vi "Kinect Acquire.vi"(8 "error in":errorcluster, 11 "Queue in":refnum<queue>) -> (0 "error out":errorcluster, 1 "Timestamp":i32, 2 "Difference\nImage":T1(plugin-control), 3 "Image Out":T1(plugin-control))   [LabVIEW 2011]
uses:
  Kinect Data Cluster.ctl
  <vilib>/vision/NI_Vision_Development_Module.lvlib
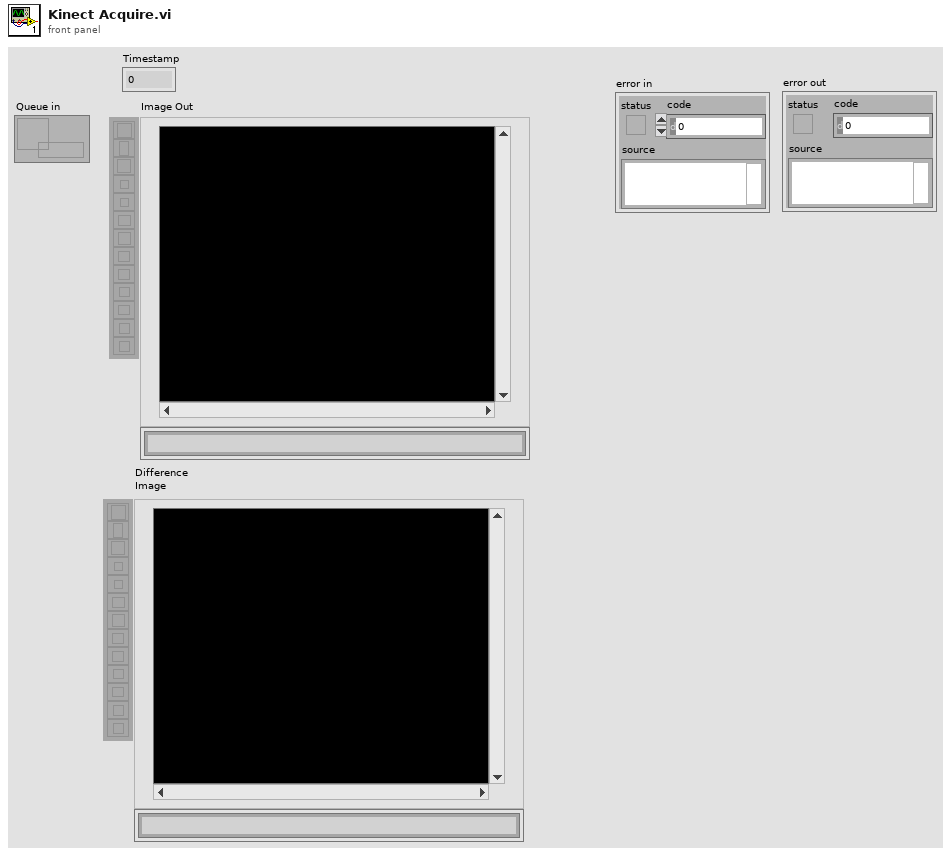
[diagram p1: front panel]
types:
  T1 = typedef "IMAQ Image.ctl" = refnum<image>
  T2 = typedef "Image Type" = u32
  T3 = typedef "Kinect Data Cluster.ctl" = cluster{"1D Depth Data":i16[], "Width":i32, "Height":i32, "Timestamp":i32}
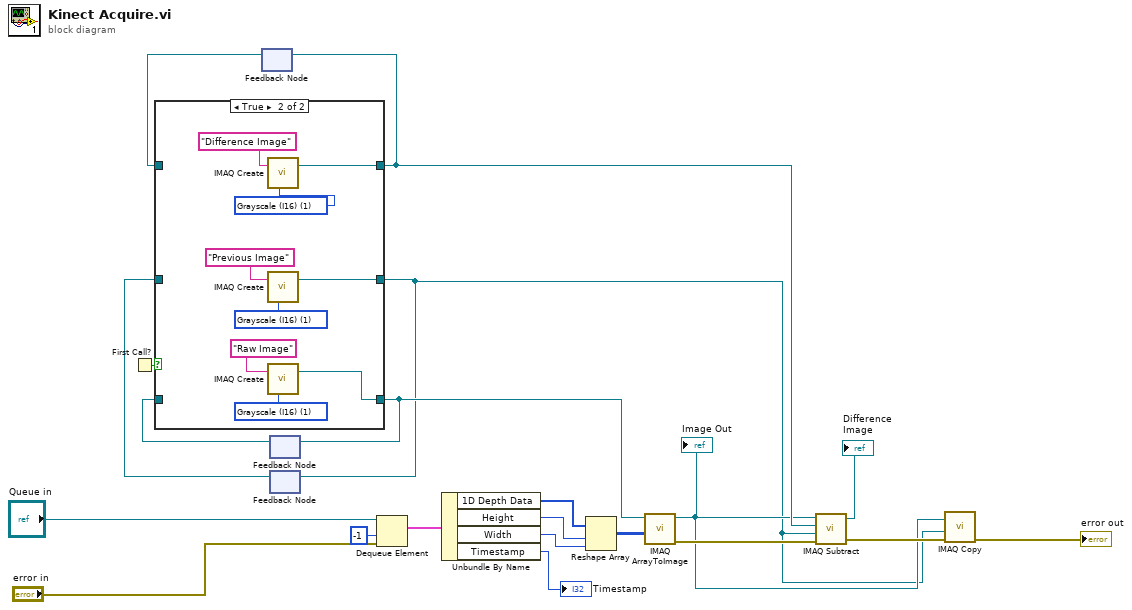
[diagram p0: block diagram]
diagram:
  n1 = First Call?() -> (First Call?: T/F=w8:bool)
  n2 = feedback #1() -> (w16:T1)  [unwired: 1 in]
  n3 = feedback #2() -> (w10:T1)  [unwired: 1 in]
  n4 = feedback #3() -> (w20:T1)  [unwired: 1 in]
  n5 = case shown="True" w8 {
    tunnel: [w24 w31] -> w9
    tunnel: w10 -> [w24 _]
    tunnel: [w23 w29] -> w17
    tunnel: w16 -> [w23 _]
    tunnel: [w22 w25] -> w3
    tunnel: w20 -> [w22 _]
    frame False {
    }
    frame True {
      w27 = T2 1 items=["Grayscale (U8)", "Grayscale (I16)", "Grayscale (SGL)", "Complex (CSG)", "RGB (U32)", "HSL (U32)", "RGB (U64)", "Grayscale (U16)"] ("Image Type")
      w28 = T2 1 items=["Grayscale (U8)", "Grayscale (I16)", "Grayscale (SGL)", "Complex (CSG)", "RGB (U32)", "HSL (U32)", "RGB (U64)", "Grayscale (U16)"] ("Image Type")
      w32 = T2 1 items=["Grayscale (U8)", "Grayscale (I16)", "Grayscale (SGL)", "Complex (CSG)", "RGB (U32)", "HSL (U32)", "RGB (U64)", "Grayscale (U16)"] ("Image Type")
      n6 = call "IMAQ Create"("Image Name"="Difference Image", "Image Type"=w28) -> ("New Image"=w29:T1)  [unwired: 3 in, 1 out]
      n7 = call "IMAQ Create"("Image Name"="Previous Image", "Image Type"=w27) -> ("New Image"=w25:T1)  [unwired: 3 in, 1 out]
      n8 = call "IMAQ Create"("Image Name"="Raw Image", "Image Type"=w32) -> ("New Image"=w31:T1)  [unwired: 3 in, 1 out]
    }
  }
  n9 = feedback-in #1(w17) -> ()
  n10 = feedback-in #2(w9) -> ()
  n11 = feedback-in #3(w3) -> ()
  n12 = Dequeue Element(queue="Queue in", timeout in ms (-1)=-1, error in (no error)="error in") -> (element=w12:T3)  [unwired: 3 out]
  n13 = Unbundle By Name(w12) -> ("1D Depth Data"=w13:i16[], "Height"=w14:i32, "Width"=w15:i32, "Timestamp"=→"Timestamp":i32)
  n14 = Reshape Array(w13, w14, w15) -> (w7:i16[][])
  n15 = call "IMAQ ArrayToImage"("Image Pixels (I16)"=w7, "Image"=w9) -> ("error out"=w18:errorcluster, "Image Out"=w4:T1)  [unwired: 8 in]
  "Image Out" <- w4
  n16 = call "IMAQ Subtract"("Image Src A"=w4, "Image Dst"=w17, "Image Src B"=w3, "error in (no error)"=w18) -> ("Image Dst Out"=→"Difference\nImage":T1, "error out"=w5:errorcluster)  [unwired: 3 in]
  n17 = call "IMAQ Copy"("error in (no error)"=w5, "Image Dst"=w3, "Image Src"=w4) -> ("error out"=→"error out":errorcluster)  [unwired: 3 in, 1 out]
